vi "Add topic to topics.vi"(10 "Topic":string, 11 "EHL DATA in":T1) -> (3 "EHL DATA out":T1)   [LabVIEW 2016, in "MQTT_Client.lvlib"]
uses:
  MQTT_Client.lvlib
  Module Data EHL--cluster.ctl
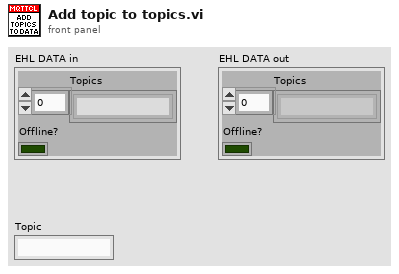
[diagram p1: front panel]
types:
  T1 = typedef "MQTT_Client.lvlib/Module Data EHL--cluster.ctl" = cluster{"Topics":string[], "Offline?":bool}
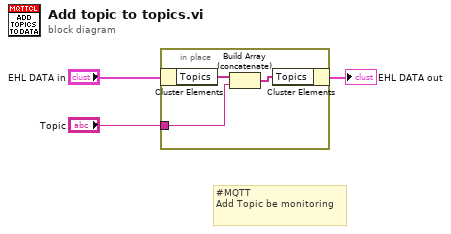
[diagram p0: block diagram]
diagram:
  # "#MQTT   \nAdd Topic be monitoring"
  n1 = in-place {
    in-place-border: "Topic" -> [w5]
    n2 = in-place-cluster #1("EHL DATA in") -> ("Topics"=w6:string[])
    n3 = Build Array (concatenate)(w6, w5) -> (w4:string[])
    n4 = in-place-cluster #1("Topics"=w4) -> (→"EHL DATA out":T1)
  }
